vi "wsp_korelacji.vi"() -> ()   [LabVIEW 2025]
panel:
  out "f_corr":dbl
  in  "m":dbl
  out "kowariancja":dbl
  out "korelacja":dbl
  in  "Amp 2":dbl
  in  "Sygnal 2":T1(ring)
  in  "phase 2":dbl
  in  "liczba cykli 2":i64
  in  "samples":i32=128
  in  "Amp":dbl
  in  "Sygnal":T1(ring)
  in  "phase":dbl
  in  "liczba cykli":i64
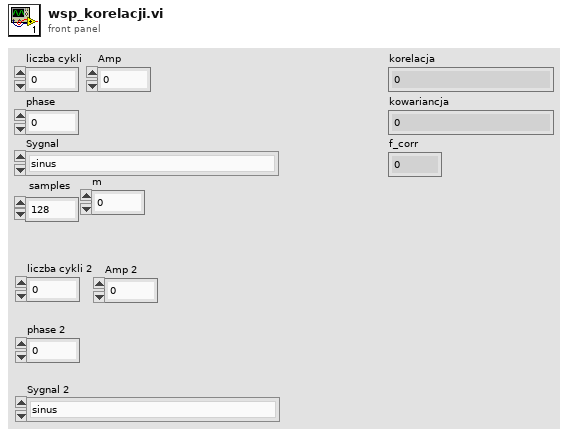
[diagram p1: front panel]
types:
  T1 = enum16{"sinus", "prostokat", "pila", "trojkat", "rozklad losowy", "rozklad normalny"}
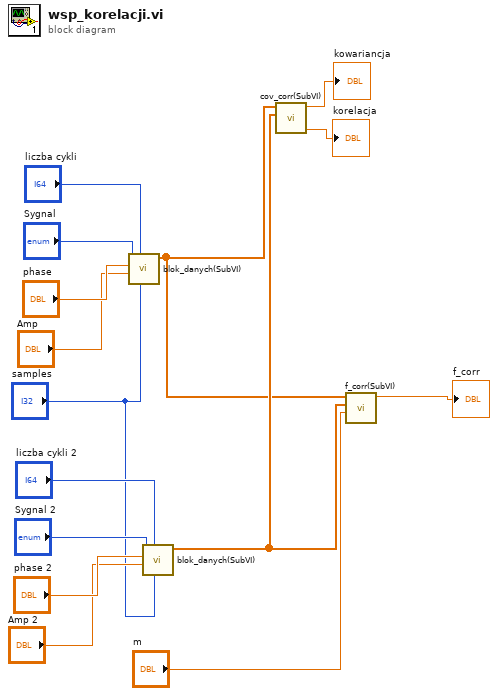
[diagram p0: block diagram]
diagram:
  n1 = call "blok_danych(SubVI).vi"("samples"="samples", "liczba cykli"="liczba cykli", "Amp"="Amp", "phase"="phase", "Sygnal"="Sygnal") -> ("Gaussian noise pattern"=w2:dbl[])  [unwired: 6 in]
  n2 = call "blok_danych(SubVI).vi"("samples"="samples", "liczba cykli"="liczba cykli 2", "Amp"="Amp 2", "phase"="phase 2", "Sygnal"="Sygnal 2") -> ("Gaussian noise pattern"=w4:dbl[])  [unwired: 6 in]
  n3 = call "cov_corr(SubVI).vi"("Gaussian noise pattern 2"=w4, "Gaussian noise pattern"=w2) -> ("korelacja"=→"korelacja":dbl, "kowariancja"=→"kowariancja":dbl)  [unwired: 8 in]
  n4 = call "f_corr(SubVI).vi"("m"="m", "Gaussian noise pattern 2"=w4, "Gaussian noise pattern"=w2) -> ("f_corr"=→"f_corr":dbl)  [unwired: 8 in]
